vi "close-camera-file.vi"(11 "ir_file_handler":u64) -> (3 "return type":i32)   [LabVIEW 2011, in "librir.lvlib"]
uses:
  librir.lvlib
  libs/video_io.dll
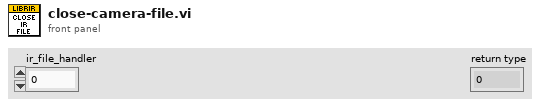
[diagram p1: front panel]
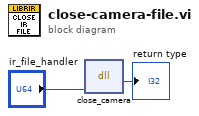
[diagram p0: block diagram]
diagram:
  n1 = dll-call lib="G:/librir/src/labview/libs/video_io.dll" fn="close_camera"("ir_file_handler"="ir_file_handler") -> ("return type"=→"return type":i32)  [unwired: 4 in, 2 out]
